vi "parseReportServerStatusFrame.vi"(8 "error in (no error)":errorcluster, 10 "ModbusBuffer in":refnum<class "ModbusBuffer.lvclass">, 11 "ILC in":refnum<class "ILC.lvclass">) -> (0 "error out":errorcluster, 2 "ModbusBuffer out":refnum<class "ModbusBuffer.lvclass">, 3 "ILC out":refnum<class "ILC.lvclass">)   [LabVIEW 2016, in "RTILC.lvlib" / "ILC.lvclass"]
uses:
  ILC.lvclass
  Common_RT_Modbus/ModbusBuffer/ModbusBuffer.lvclass
  Common_RT_Modbus/ModbusBuffer/ModbusBuffer.lvclass/ModbusBuffer.ctl
  Common_RT_Modbus/DataTypes/ExceptionCodes.ctl
  ILC.lvclass/ILC.ctl
  Common_RT_Modbus/ModbusBuffer/readTimestampByte.vi
  Common_RT_Modbus/ModbusBuffer/readInstructionByte.vi
  Common_RT_Modbus/RTModbus.lvlib
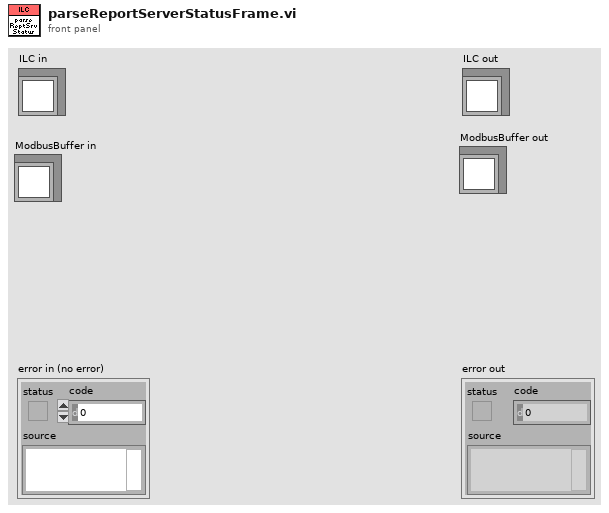
[diagram p1: front panel]
types:
  T1 = typedef "RTModbus.lvlib/ExceptionCodes.ctl" = u16
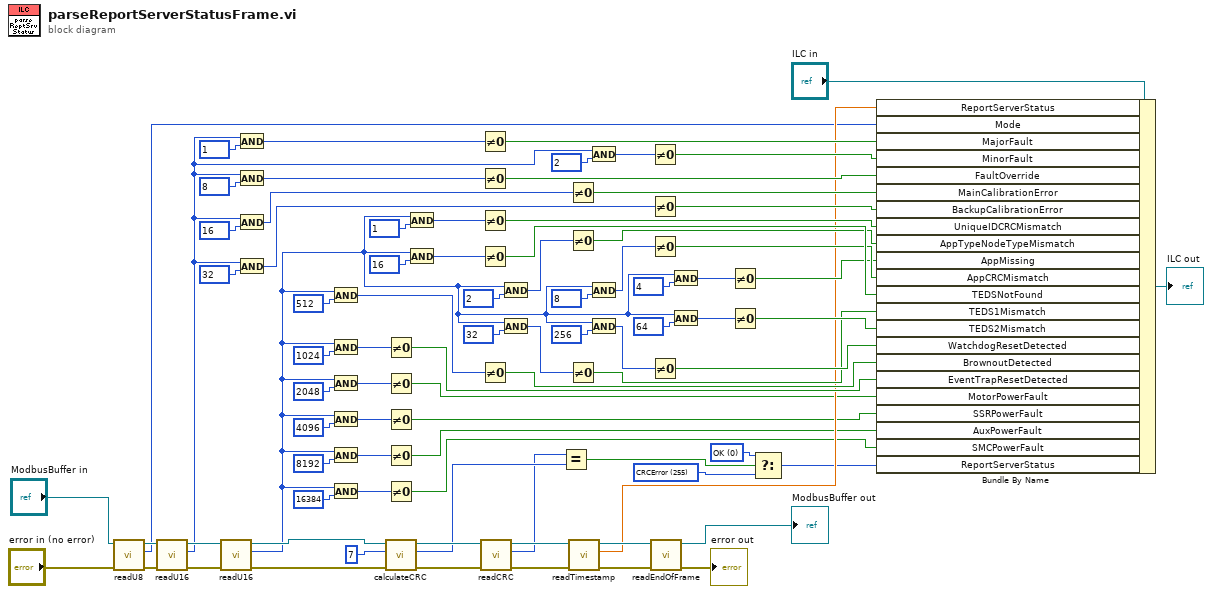
[diagram p0: block diagram]
diagram:
  w37 = T1 255 items=["OK"=0, "IllegalFunction"=1, "IllegalDataAddress"=2, "IllegalDataValue"=3, "SlaveDeviceFailure"=4, "Acknowledge"=5, "SlaveDeviceBusy"=6, "NegativeAcknowledge"=7, "MemoryParityError"=8, "GatewayPathUnavailable"=9, "GatewayTargetDeviceFailedToRespond"=10, "WaitingForResponse"=254, "CRCError"=255] ("f")
  w38 = T1 0 items=["OK"=0, "IllegalFunction"=1, "IllegalDataAddress"=2, "IllegalDataValue"=3, "SlaveDeviceFailure"=4, "Acknowledge"=5, "SlaveDeviceBusy"=6, "NegativeAcknowledge"=7, "MemoryParityError"=8, "GatewayPathUnavailable"=9, "GatewayTargetDeviceFailedToRespond"=10, "WaitingForResponse"=254, "CRCError"=255] ("Responses.ADCOffsetSensitivity")
  n1 = call "readU8.vi"("error in (no error)"="error in (no error)", "ModbusBuffer in"="ModbusBuffer in") -> ("error out"=w21:errorcluster, "Output"=w16:u8, "ModbusBuffer out"=w25:refnum<class "ModbusBuffer.lvclass">)  [unwired: 7 in]
  n2 = call "readU16.vi"("error in (no error)"=w21, "ModbusBuffer in"=w25) -> ("error out"=w20:errorcluster, "Output"=w15:u16, "ModbusBuffer out"=w24:refnum<class "ModbusBuffer.lvclass">)  [unwired: 7 in]
  n3 = call "readU16.vi"("error in (no error)"=w20, "ModbusBuffer in"=w24) -> ("error out"=w19:errorcluster, "Output"=w5:u16, "ModbusBuffer out"=w23:refnum<class "ModbusBuffer.lvclass">)  [unwired: 7 in]
  n4 = And(x=w15, y=u16 1) -> (x .and. y?=w51:u16)
  n5 = And(x=w15, y=u16 8) -> (x .and. y?=w53:u16)
  n6 = And(x=w15, y=u16 16) -> (x .and. y?=w43:u16)
  n7 = And(x=w15, y=u16 32) -> (x .and. y?=w42:u16)
  n8 = And(x=w5, y=u16 512) -> (x .and. y?=w58:u16)
  n9 = And(x=w5, y=u16 1024) -> (x .and. y?=w57:u16)
  n10 = And(x=w5, y=u16 2048) -> (x .and. y?=w13:u16)
  n11 = And(x=w5, y=u16 4096) -> (x .and. y?=w10:u16)
  n12 = And(x=w5, y=u16 8192) -> (x .and. y?=w9:u16)
  n13 = And(x=w5, y=u16 16384) -> (x .and. y?=w6:u16)
  n14 = Not Equal To 0?(x=w57) -> (x != 0?=w86:bool)
  n15 = Not Equal To 0?(x=w13) -> (x != 0?=w4:bool)
  n16 = Not Equal To 0?(x=w10) -> (x != 0?=w3:bool)
  n17 = Not Equal To 0?(x=w9) -> (x != 0?=w2:bool)
  n18 = Not Equal To 0?(x=w6) -> (x != 0?=w1:bool)
  n19 = call "calculateCRC.vi"("error in (no error)"=w19, "Length"=u16 7, "ModbusBuffer in"=w23) -> ("error out"=w31:errorcluster, "CRC"=w30:u16, "ModbusBuffer out"=w36:refnum<class "ModbusBuffer.lvclass">)  [unwired: 6 in]
  n20 = And(x=w5, y=u16 1) -> (x .and. y?=w66:u16)
  n21 = And(x=w5, y=u16 16) -> (x .and. y?=w62:u16)
  n22 = Not Equal To 0?(x=w51) -> (x != 0?=w54:bool)
  n23 = Not Equal To 0?(x=w53) -> (x != 0?=w56:bool)
  n24 = Not Equal To 0?(x=w66) -> (x != 0?=w77:bool)
  n25 = Not Equal To 0?(x=w62) -> (x != 0?=w81:bool)
  n26 = Not Equal To 0?(x=w58) -> (x != 0?=w85:bool)
  n27 = call "readCRC.vi"("error in (no error)"=w31, "ModbusBuffer in"=w36) -> ("error out"=w32:errorcluster, "Output"=w29:u16, "ModbusBuffer out"=w35:refnum<class "ModbusBuffer.lvclass">)  [unwired: 7 in]
  n28 = And(x=w5, y=u16 2) -> (x .and. y?=w65:u16)
  n29 = And(x=w5, y=u16 32) -> (x .and. y?=w61:u16)
  n30 = Equal?(x=w29, y=w30) -> (x = y?=w39:bool)
  n31 = Not Equal To 0?(x=w43) -> (x != 0?=w41:bool)
  n32 = Not Equal To 0?(x=w65) -> (x != 0?=w78:bool)
  n33 = Not Equal To 0?(x=w61) -> (x != 0?=w82:bool)
  n34 = call "readTimestamp.vi"("error in (no error)"=w32, "ModbusBuffer in"=w35) -> ("error out"=w33:errorcluster, "Output"=w17:dbl, "ModbusBuffer out"=w34:refnum<class "ModbusBuffer.lvclass">)  [unwired: 7 in]
  n35 = And(x=w15, y=u16 2) -> (x .and. y?=w52:u16)
  n36 = And(x=w5, y=u16 8) -> (x .and. y?=w63:u16)
  n37 = And(x=w5, y=u16 256) -> (x .and. y?=w59:u16)
  n38 = Not Equal To 0?(x=w52) -> (x != 0?=w55:bool)
  n39 = Not Equal To 0?(x=w42) -> (x != 0?=w40:bool)
  n40 = Not Equal To 0?(x=w63) -> (x != 0?=w80:bool)
  n41 = Not Equal To 0?(x=w59) -> (x != 0?=w84:bool)
  n42 = call "readEndOfFrame.vi"("error in (no error)"=w33, "ModbusBuffer in"=w34) -> ("error out"=→"error out":errorcluster, "ModbusBuffer out"=→"ModbusBuffer out":refnum<class "ModbusBuffer.lvclass">)  [unwired: 8 in]
  n43 = And(x=w5, y=u16 4) -> (x .and. y?=w64:u16)
  n44 = And(x=w5, y=u16 64) -> (x .and. y?=w60:u16)
  n45 = Not Equal To 0?(x=w64) -> (x != 0?=w79:bool)
  n46 = Not Equal To 0?(x=w60) -> (x != 0?=w83:bool)
  n47 = Select(t=w38, s=w39, f=w37) -> (s? t:f=w14:T1)
  n48 = Bundle By Name(cluster="ILC in", "ReportServerStatus"=w17, "Mode"=w16, "MajorFault"=w54, "MinorFault"=w55, "FaultOverride"=w56, "MainCalibrationError"=w41, "BackupCalibrationError"=w40, "UniqueIDCRCMismatch"=w77, "AppTypeNodeTypeMismatch"=w78, "AppMissing"=w79, "AppCRCMismatch"=w80, "TEDSNotFound"=w81, "TEDS1Mismatch"=w82, "TEDS2Mismatch"=w83, "WatchdogResetDetected"=w84, "BrownoutDetected"=w85, "EventTrapResetDetected"=w86, "MotorPowerFault"=w4, "SSRPowerFault"=w3, "AuxPowerFault"=w2, "SMCPowerFault"=w1, "ReportServerStatus"=w14) -> (→"ILC out":refnum<class "ILC.lvclass">)
